vi "VNA_ConfigureTraces.vi"(0 "VISA resource name":refnum<visa-resource-name>, 1 "Def 2":T1(ring), 2 "Def 1":T1(ring), 3 "Def 3":T1(ring), 4 "Def 4":T1(ring), 5 "error in (no error)":errorcluster, 7 "Data Format (0: Logaritmic Magnitude)":u16(ring) items=["Logaritmic Magnitude", "Phase", "Group Delay", "Smith Chart  Linear (Lin/Phase)", "Smith Chart  Logaritmic (Log/Phase)", "Smith Chart  Complex (Real/Imag)", "Smith Chart  Impedance (R+jX)", "Smith Chart  Admittance (G+jB)", "Polar Format (Linear)", "Polar Format (Logaritmic)", "Polar Format (Re/Im)", "Linear Magnitude", "SWR", "Real", "Imaginary", "Epanded Phase", "Positive Phase"]) -> (6 "VISA VNA out":refnum<visa-resource-name>, 8 "error out":errorcluster)   [LabVIEW 2017]
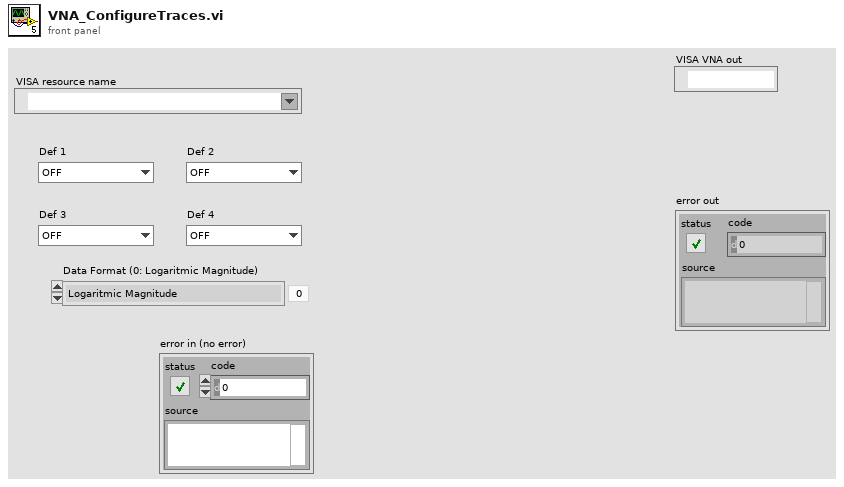
[diagram p1: front panel]
types:
  T1 = enum16{"OFF", "S11", "S21", "S12", "S22", "A", "B", "C", "D", "R1", "R2", "AUX1", "AUX2"}
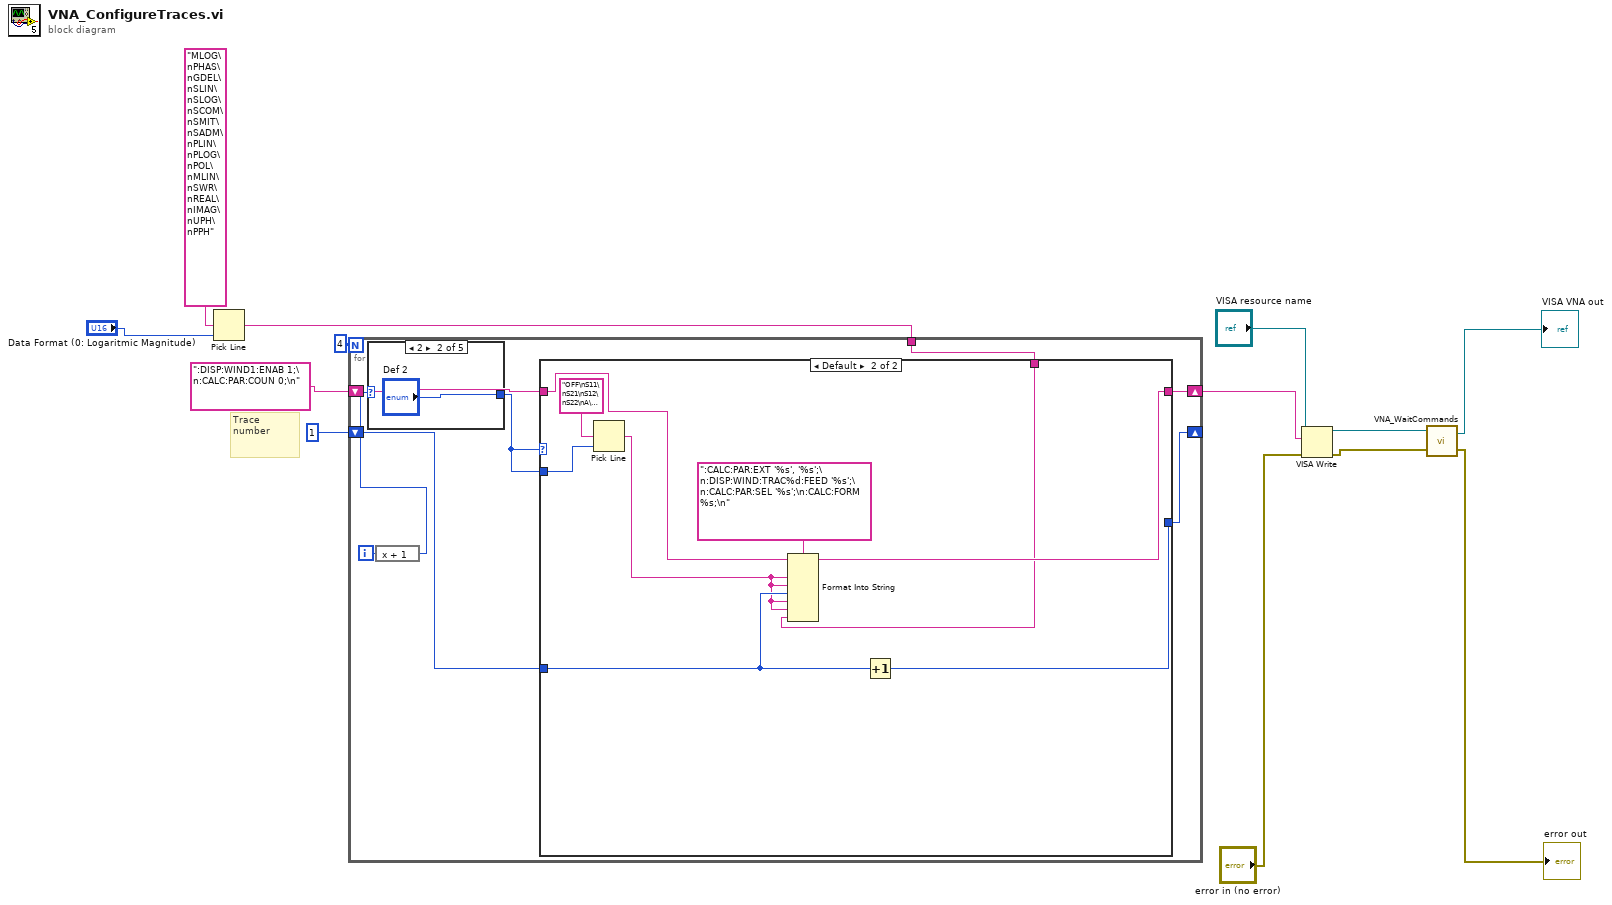
[diagram p0: block diagram]
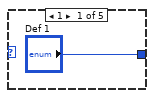
[diagram p3: hidden frame]
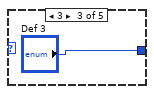
[diagram p4: hidden frame]
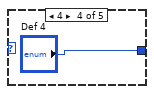
[diagram p5: hidden frame]
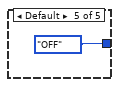
[diagram p6: hidden frame]
diagram:
  # "Trace number"
  n1 = Pick Line(multi-line string="MLOG\nPHAS\nGDEL\nSLIN\nSLOG\nSCOM\nSMIT\nSADM\nPLIN\nPLOG\nPOL\nMLIN\nSWR\nREAL\nIMAG\nUPH\nPPH" ("string (\"\")"), line index="Data Format (0: Logaritmic Magnitude)") -> (output string=w9:string)  [unwired: 1 in]
  n2 = for {
    N: 4 -> [_]
    shift-right: [w15] -> w3
    shift-left: ":DISP:WIND1:ENAB 1;\n:CALC:PAR:COUN 0;\n" -> [w16]
    tunnel: w9 -> [w14]
    shift-right: [w18] -> _
    shift-left: 1 -> [w19]
    i -> [w21]
    n3 = expression code="x + 1"(w21) -> (w20:i32)
    n4 = case shown="2" w20 {
      tunnel: ["Def 1" "Def 2" "Def 3" "Def 4" T1."OFF" ("Def 4")] -> w17
      frame 1 {
      }
      frame 2 {
      }
      frame 3 {
      }
      frame 4 {
      }
      frame Default {
      }
    }
    n5 = case shown="Default" w17 {
      tunnel: w17 -> [_ w31]
      tunnel: [w23 w30] -> w18
      tunnel: w19 -> [w23 w27]
      tunnel: w16 -> [w22 w28]
      tunnel: [w22 w26] -> w15
      tunnel: w14 -> [_ w24]
      frame "OFF" {
      }
      frame Default {
        n6 = Pick Line(multi-line string="OFF\nS11\nS21\nS12\nS22\nA\nB\nC\nD\nR1\nR2\nAUX1\nAUX2", line index=w31) -> (output string=w25:string)  [unwired: 1 in]
        n7 = Format Into String(format string=":CALC:PAR:EXT '%s', '%s';\n:DISP:WIND:TRAC%d:FEED '%s';\n:CALC:PAR:SEL '%s';\n:CALC:FORM %s;\n", initial string=w28, w25, w25, w27, w25, w25, w24) -> (resulting string=w26:string)  [unwired: 1 in, 1 out]
        n8 = Increment(x=w27) -> (x+1=w30:i32)
      }
    }
  }
  n9 = VISA Write(VISA resource name="VISA resource name", write buffer=w3, error in (no error)="error in (no error)") -> (VISA resource name out=w7:refnum<visa-resource-name>, error out=w6:errorcluster)  [unwired: 1 out]
  n10 = call "VNA_WaitCommands.vi"("error in (no error)"=w6, "VISA resource name"=w7) -> ("error out"=→"error out":errorcluster, "VISA resource name out"=→"VISA VNA out":refnum<visa-resource-name>)
